vi "CleanUp.vi"(0 "object in":refnum<class "InterceptBallTactic.lvclass">, 5 "error in (no error)":errorcluster) -> (14 "object out":refnum<class "InterceptBallTactic.lvclass">, 19 "error out":errorcluster)   [LabVIEW 2023, in "InterceptBallTactic.lvclass"]
uses:
  InterceptBallTactic.lvclass
  NewSTP/NewTactics/Tactic_v2_class/Tactic_v2.lvclass
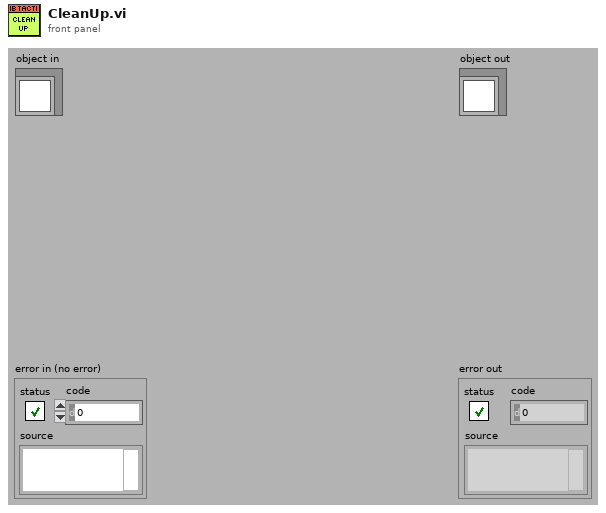
[diagram p1: front panel]
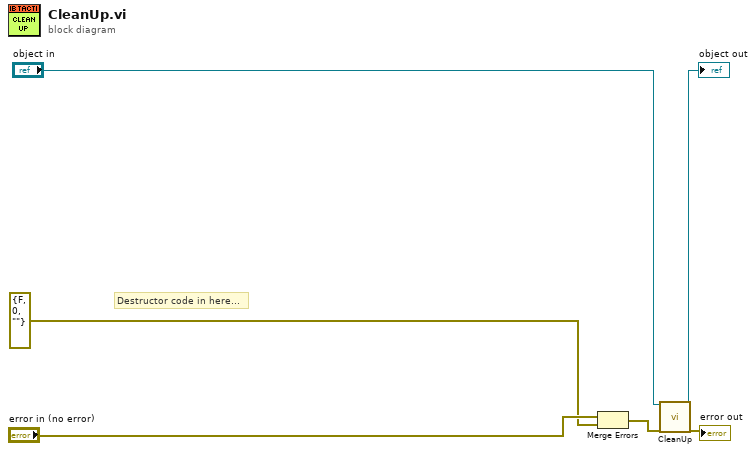
[diagram p0: block diagram]
diagram:
  # "Destructor code in here..."
  n1 = Merge Errors("error in (no error)", errorcluster {"status"=FALSE, "code"=0, "source"=""} ("error in (no error)")) -> (w2:errorcluster)
  n2 = call-parent "CleanUp.vi"("object in"="object in", "error in (no error)"=w2) -> ("object out"=→"object out":refnum<class "InterceptBallTactic.lvclass">, "error out"=→"error out":errorcluster)  [unwired: 16 in]
